vi "Convert XY to polar graph.vi"(2 "Y":cluster{"Y":dbl[], "Y":dbl[]}[](array[cluster]), 3 "X":cluster{"Y":dbl[], "Y":dbl[]}[](array[cluster])) -> (0 "Array":cluster{"Y":dbl[], dbl[]}[](array[cluster]), 1 "Array 2":cluster{"Y":dbl[], dbl[]}[](array[cluster]))   [LabVIEW 2016]
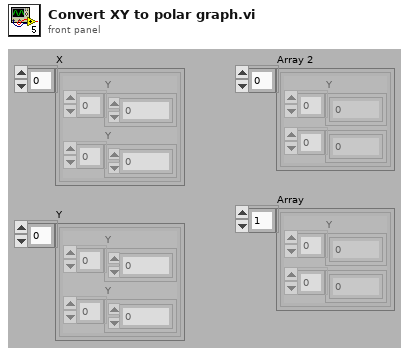
[diagram p1: front panel]
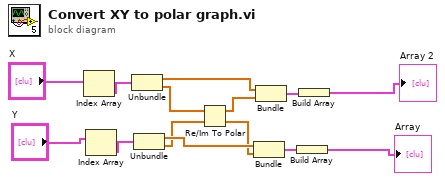
[diagram p0: block diagram]
diagram:
  n1 = Index Array(array="X") -> (element=w2:cluster{"Y":dbl[], "Y":dbl[]})  [unwired: 1 in]
  n2 = Index Array(array="Y") -> (element=w3:cluster{"Y":dbl[], "Y":dbl[]})  [unwired: 1 in]
  n3 = Unbundle(w2) -> ("Y"=w8:dbl[], "Y"=w5:dbl[])
  n4 = Unbundle(w3) -> ("Y"=w10:dbl[], "Y"=w6:dbl[])
  n5 = Re/Im To Polar(2:w6, 3:w5) -> (0:w9:dbl[], 1:w7:dbl[])
  n6 = Bundle("Y"=w10, w9) -> (w12:cluster{"Y":dbl[], dbl[]})  [unwired: 1 in]
  n7 = Bundle("Y"=w8, w7) -> (w11:cluster{"Y":dbl[], dbl[]})  [unwired: 1 in]
  n8 = Build Array(w12) -> (→"Array":cluster{"Y":dbl[], dbl[]}[])
  n9 = Build Array(w11) -> (→"Array 2":cluster{"Y":dbl[], dbl[]}[])
